vi "MessageRecieved.vi"(8 "error in (no error)":errorcluster, 10 "clientMessage":T1, 11 "TCP_Server in":refnum<class "TCP_Server.lvclass">) -> (0 "error out":errorcluster, 3 "TCP_Server out":refnum<class "TCP_Server.lvclass">)   [LabVIEW 2023, in "TCP_Server.lvlib" / "TCP_Server.lvclass"]
uses:
  TCP_Server.lvclass
  C:/Program Files (x86)/National Instruments/LabVIEW 2023/vi.lib/ActorFramework/Actor/Actor.lvclass
  TCP_Server_Connection_Handler/TypeDefinitions/ClientMessage.ctl
  TCP_Server.lvclass/TCP_Server.ctl
  TCP_Client_Window/TCP_Client_Window Messages/NewClientMessage Msg/NewClientMessage Msg.lvclass/NewClientMessage Msg.ctl
  <vilib>/ActorFramework/Message Enqueuer/Message Enqueuer.lvclass/Message Enqueuer.ctl
  <vilib>/ActorFramework/Actor/Actor.lvclass/Actor.ctl
  <vilib>/ActorFramework/Message Enqueuer/Enqueue.vi
  <vilib>/ActorFramework/Message Enqueuer/Init from Existing Queue.vi
  TCP_Client_Window/TCP_Client_Window Messages/NewClientMessage Msg/NewClientMessage Msg.lvclass
  C:/Program Files (x86)/National Instruments/LabVIEW 2023/vi.lib/ActorFramework/Message/Message.lvclass
  <vilib>/ActorFramework/Stop Msg/Stop Msg.lvclass
  <vilib>/ActorFramework/Message Priority Queue/Priority Enqueue.vi
  <vilib>/ActorFramework/Message Enqueuer/Message Enqueuer.lvclass
  <vilib>/ActorFramework/Actor/Actor.lvclass
  TCP_Server_Connection_Handler/TCP_Server_Connection_Handler.lvlib
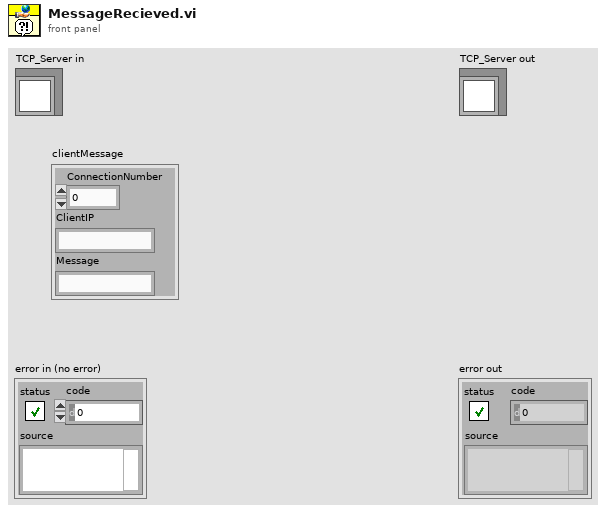
[diagram p1: front panel]
types:
  T1 = typedef "TCP_Server_Connection_Handler.lvlib/ClientMessage.ctl" = cluster{"ConnectionNumber":i32, "ClientIP":string, "Message":string}
  T2 = typedef "TCP_Server.lvlib/ServerConnection.ctl" = cluster{"Connection Handlers's Enqueuer":refnum<class "Message Enqueuer.lvclass">, "Connection Window's Enqueuer":refnum<class "Message Enqueuer.lvclass">, "Connection Information":T3}
  T3 = typedef "TCP_Listener.lvlib/ConnectionInformation.ctl" = cluster{"Connection number":i32, "Remote Address":string, "Remote Port":u16, "Connection ID":refnum<k5>}
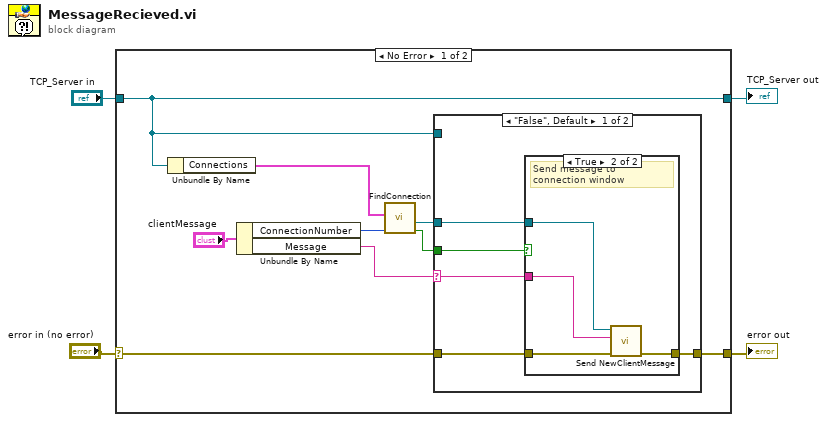
[diagram p0: block diagram]
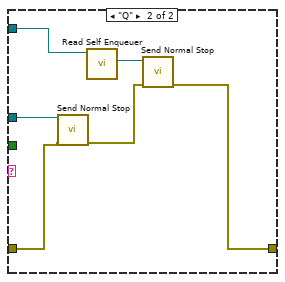
[diagram p3: hidden frame]
diagram:
  n1 = case shown="No Error" "error in (no error)" {
    selector: "error in (no error)" -> [w12 w31]
    tunnel: [w11 w31] -> w3
    tunnel: "TCP_Server in" -> [w10 w30]
    tunnel: [w10 w30] -> w1
    frame No Error {
      n2 = Unbundle By Name(w10) -> ("Connections"=w5:T2[])
      n3 = Unbundle By Name("clientMessage") -> ("ConnectionNumber"=w8:i32, "Message"=w9:string)
      n4 = call "FindConnection.vi"("Connection number"=w8, "Connections"=w5) -> ("Found?"=w7:bool, "Connection Window's Enqueuer"=w6:refnum<class "Message Enqueuer.lvclass">)  [unwired: 6 in, 2 out]
      n5 = case shown="\"False\", Default" w9 {
        selector: w9 -> [w18 _]
        tunnel: w12 -> [w17 w26]
        tunnel: [w16 w24] -> w11
        tunnel: w10 -> [_ w29]
        tunnel: w7 -> [w15 _]
        tunnel: w6 -> [w14 w27]
        frame "False", Default {
          n6 = case shown="True" w15 {
            tunnel: w18 -> [_ w23]
            tunnel: w17 -> [w19 w22]
            tunnel: [w19 w21] -> w16
            tunnel: w14 -> [_ w20]
            frame False {
              # "connection not found"
            }
            frame True {
              # "Send message to connection window"
              n7 = call "Send NewClientMessage.vi"("error in (no error)"=w22, "Message from client"=w23, "Message Enqueuer"=w20) -> ("error out"=w21:errorcluster)  [unwired: 7 in, 1 out]
            }
          }
        }
        frame "Q" {
          n8 = call <vilib>:"Send Normal Stop.vi"("error in (no error)"=w26, "Message Enqueuer"=w27) -> ("error out"=w25:errorcluster)  [unwired: 9 in]
          n9 = call <vilib>:"Read Self Enqueuer.vi"("Actor"=w29) -> ("Self Enqueuer"=w28:refnum<class "Message Enqueuer.lvclass">)  [unwired: 10 in]
          n10 = call <vilib>:"Send Normal Stop.vi"("error in (no error)"=w25, "Message Enqueuer"=w28) -> ("error out"=w24:errorcluster)  [unwired: 9 in]
        }
      }
    }
    frame Error {
    }
  }
  "error out" <- w3
  "TCP_Server out" <- w1
